vi "HRM-Stage4-close_main.vi"(8 "error in (no error)":errorcluster, 11 "Init cluster":T1) -> (0 "error out":errorcluster)   [LabVIEW 2020]
uses:
  HRM-Stage4-init_cluster.ctl
  HRM-stage4-config_data.ctl
  HRM-Stage4-User_events.ctl
  process/HRM-process-peak_detect_setting.ctl
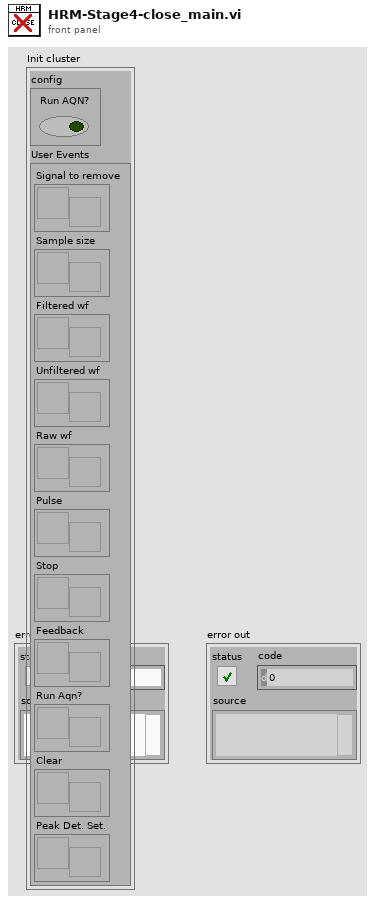
[diagram p1: front panel]
types:
  T1 = typedef "HRM-Stage4-init_cluster.ctl" = cluster{"config":T2, "User Events":T3}
  T2 = typedef "HRM-stage4-config_data.ctl" = cluster{"Run AQN?":bool}
  T3 = typedef "HRM-Stage4-User_events.ctl" = cluster{"Signal to remove":refnum<user-event>, "Sample size":refnum<user-event>, "Filtered wf":refnum<user-event>, "Unfiltered wf":refnum<user-event>, "Raw wf":refnum<user-event>, "Pulse":refnum<user-event>, "Stop":refnum<user-event>, "Feedback":refnum<user-event>, "Run Aqn?":refnum<user-event>, "Clear":refnum<user-event>, "Peak Det. Set.":refnum<user-event>}
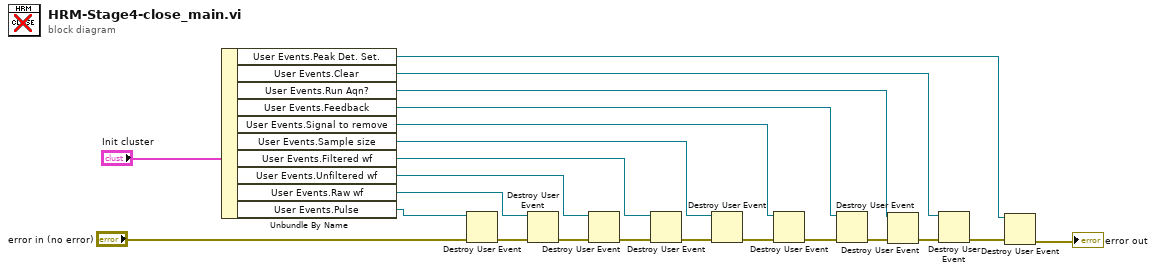
[diagram p0: block diagram]
diagram:
  n1 = Unbundle By Name("Init cluster") -> ("User Events.Peak Det. Set."=w2:refnum<user-event>, "User Events.Clear"=w4:refnum<user-event>, "User Events.Run Aqn?"=w6:refnum<user-event>, "User Events.Feedback"=w9:refnum<user-event>, "User Events.Signal to remove"=w21:refnum<user-event>, "User Events.Sample size"=w20:refnum<user-event>, "User Events.Filtered wf"=w19:refnum<user-event>, "User Events.Unfiltered wf"=w18:refnum<user-event>, "User Events.Raw wf"=w17:refnum<user-event>, "User Events.Pulse"=w16:refnum<user-event>)
  n2 = Destroy User Event(user event=w16, error in="error in (no error)") -> (error out=w15:errorcluster)
  n3 = Destroy User Event(user event=w17, error in=w15) -> (error out=w11:errorcluster)
  n4 = Destroy User Event(user event=w18, error in=w11) -> (error out=w12:errorcluster)
  n5 = Destroy User Event(user event=w19, error in=w12) -> (error out=w13:errorcluster)
  n6 = Destroy User Event(user event=w20, error in=w13) -> (error out=w14:errorcluster)
  n7 = Destroy User Event(user event=w21, error in=w14) -> (error out=w10:errorcluster)
  n8 = Destroy User Event(user event=w9, error in=w10) -> (error out=w7:errorcluster)
  n9 = Destroy User Event(user event=w6, error in=w7) -> (error out=w5:errorcluster)
  n10 = Destroy User Event(user event=w4, error in=w5) -> (error out=w3:errorcluster)
  n11 = Destroy User Event(user event=w2, error in=w3) -> (error out=→"error out":errorcluster)
